vi "main.vi"   [LabVIEW 2023]
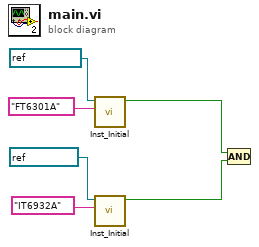
[diagram p0: block diagram]
diagram:
  n1 = call "Inst_Initial.vi"("Combo Box"="FT6301A", "VISA resource name 4"=refnum<visa-resource-name> "FT6301A") -> ("instrument ok?"=w2:bool)  [unwired: 8 in, 1 out]
  n2 = call "Inst_Initial.vi"("Combo Box"="IT6932A", "VISA resource name 4"=refnum<visa-resource-name> "IT6932A") -> ("instrument ok?"=w1:bool)  [unwired: 8 in, 1 out]
  n3 = Compound Arithmetic op=AND(w2, w1) -> ()  [unwired: 1 out]
